vi "Terminal_Gear_System_Dispaly.vi"   [LabVIEW 2014]
types:
  T1 = cluster{"油箱温度":u16, "供油油温":u16, "供油压力":u16, "油箱润滑油液位":bool, "1号油泵状态":bool, "2号油泵状态":bool, "回油泵状态":bool, "散热器风机状态":bool, "供油流量状态":bool, "过滤器压差":bool, "油箱系统综合状态":bool, "齿轮箱轴承温度1":u16, "齿轮箱轴承温度2":u16, "齿轮箱轴承温度3":u16, "齿轮箱轴承温度4":u16, "齿轮箱轴承温度5":u16, "齿轮箱轴承温度6":u16, "齿轮箱轴承温度7":u16, "齿轮箱轴承温度8":u16, "齿轮子系统状态字":cluster{"油箱加热器异常故障报警":bool, "油箱液位过高报警":bool, "油箱液位过低报警":bool, "供油过滤器压差过高报警":bool, "1号油泵故障报警":bool, "2号油泵故障报警":bool, "回油泵故障报警":bool, "散热器风机故障报警":bool, "供油压力异常报警":bool, "供油流量异常报警":bool, "供油油温异常报警":bool, "油站系统综合状态异常报警":bool, "轴承温度异常报警":bool}}
  T2 = cluster{"润滑油流量":void, "油箱润滑油液位":bool, "油箱温度":u16, "供油压力":u16, "过滤器压差":bool, "油箱液位":void, "供油油温":u16, "齿轮箱轴承温度":void, "齿轮箱高速端输出转速":void}
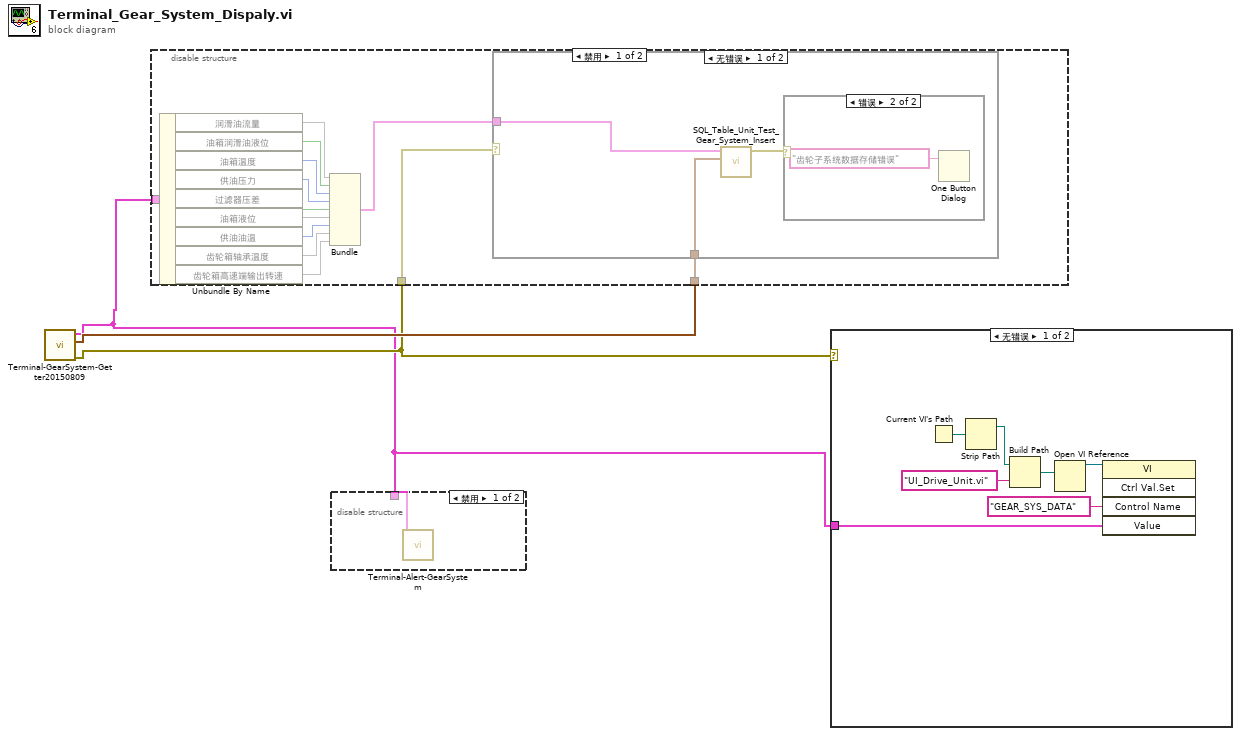
[diagram p0: block diagram]
diagram:
  n1 = call "Terminal-GearSystem-Getter20150809.vi"() -> ("error out"=w2:errorcluster, "时间标识"=w3:timestamp, "设备信息"=w1:T1)  [unwired: 9 in]
  n2 = disable-structure shown="禁用" {
    disable-tunnel: w3 -> [w6 _]
    disable-tunnel: w2 -> [w5 _]
    disable-tunnel: w1 -> [w4 _]
    frame Disabled {
      n3 = Unbundle By Name(w4) -> ("润滑油流量"=w16, "油箱润滑油液位"=w15:bool, "油箱温度"=w14:u16, "供油压力"=w13:u16, "过滤器压差"=w12:bool, "油箱液位"=w11, "供油油温"=w10:u16, "齿轮箱轴承温度"=w9, "齿轮箱高速端输出转速"=w8)
      n4 = Bundle("润滑油流量"=w16, "油箱润滑油液位"=w15, "油箱温度"=w14, "供油压力"=w13, "过滤器压差"=w12, "油箱液位"=w11, "供油油温"=w10, "齿轮箱轴承温度"=w9, "齿轮箱高速端输出转速"=w8) -> (w7:T2)  [unwired: 1 in]
      n5 = case shown="无错误" w5 {
        tunnel: w7 -> [w19 _]
        tunnel: w6 -> [w18 _]
        frame No Error {
          n6 = call "SQL_Table_Unit_Test_Gear_System_Insert.vi"("时间标识"=w18, "齿轮子系统数据"=w19) -> ("error out"=w17:errorcluster)  [unwired: 9 in]
          n7 = case shown="错误" w17 {
            frame No Error {
            }
            frame Error {
              n8 = One Button Dialog(message="齿轮子系统数据存储错误" ("消息")) -> ()  [unwired: 1 in, 1 out]
            }
          }
        }
        frame Error {
        }
      }
    }
    frame Enabled {
    }
  }
  n9 = disable-structure shown="禁用" {
    disable-tunnel: w1 -> [w21 _]
    frame Disabled {
      n10 = call "Terminal-Alert-GearSystem.vi"("齿轮子系统设备信息"=w21) -> ()  [unwired: 10 in, 1 out]
    }
    frame Enabled {
    }
  }
  n11 = case shown="无错误" w2 {
    tunnel: w1 -> [w22 _]
    frame No Error {
      n12 = Current VI's Path() -> (path=w26:path)
      n13 = Strip Path(path=w26) -> (stripped path=w27:path)  [unwired: 1 out]
      n14 = Build Path(base path=w27, name or relative path="UI_Drive_Unit.vi") -> (appended path=w24:path)
      n15 = Open VI Reference(vi path=w24) -> (vi reference=w23:refnum<vi>)  [unwired: 5 in, 1 out]
      n16 = invoke class="VI" method="Ctrl Val.Set"(reference=w23, "Control Name"="GEAR_SYS_DATA", "Value"=w22) -> ()  [unwired: 2 in, 5 out]
    }
    frame Error {
    }
  }
